vi "Ventilador2.vi"() -> ()   [LabVIEW 2019]
uses:
  <vilib>/Analysis/polynomials.llb/Polynomial Roots (DBL).vi
  <vilib>/Analysis/NI_AALPro.lvlib
panel:
  in  "Vertical Pointer Slide":dbl
  out "Aquisição pressão respiratória":dbl(graph)
  out "Válvula expiração":dbl(graph)
  in  "Pausa inspiração":dbl
  in  "Limite pressão inspiratória":dbl
  in  "OK Button":bool
  in  "Root 3":dbl
  in  "Root 2":dbl
  in  "Root 1":dbl
  in  "Incremento":dbl
  in  "Fluxo inicial":dbl
  in  "STOP":bool=TRUE
  out "Tempos de inspirações possíveis":cdb[](array[numeric])
  out "Tempo do ciclo respiratório":u32(graph)
  out "Válvula Inspiração":dbl(graph)
  in  "stop":bool
  in  "Tempo de respiração":dbl
  in  "Proporção Inspiração/respiração":string(combo)
  in  "Tempo corrido":dbl
  in  "Tipo de ventilação":string(combo)
  in  "Tipo de ciclo":string(combo)
  in  "Volume corrente":dbl
  in  "Tempo expiratório":dbl
  in  "Tempo inspiratório":dbl
  out "Fluxo respiratório medido":dbl
  in  "Frequência respiratória":dbl
  in  "Forma de onda":string(combo)
  in  "Fluxo respiratório set point":dbl
  # "rpm"
  # "(cmH2O)"
  # "(s)"
  # "\"Pausa inspiração\" neste programa está funcionando\ntambém como tempo de inspiração \ntotal, dado que não temos ainda nem \no controle nem a estimativa da rampa \nde subida da pressão do pulmão do paciente\npara diferenciar os valores"
  # "\"Vertical Pointer Slide\" está simulando a pressão\nno pulmão do paciente, você deve\n setá-lo para o valor de \"Limite pressão \ninspiratória\" quando Válvula inspiração =1 (aberta) e \nVálvula expiração = 0 (fechada) e para 0 (ou um valor \ndiferente de \"Limite pressão Inspiratória\") quando \nVálvula inspiração = 0 (fechada) e  Válvula expiração = 1 \n(aberta) para simular o ciclo de respiração natural."
  # "(s)"
  # "(s)"
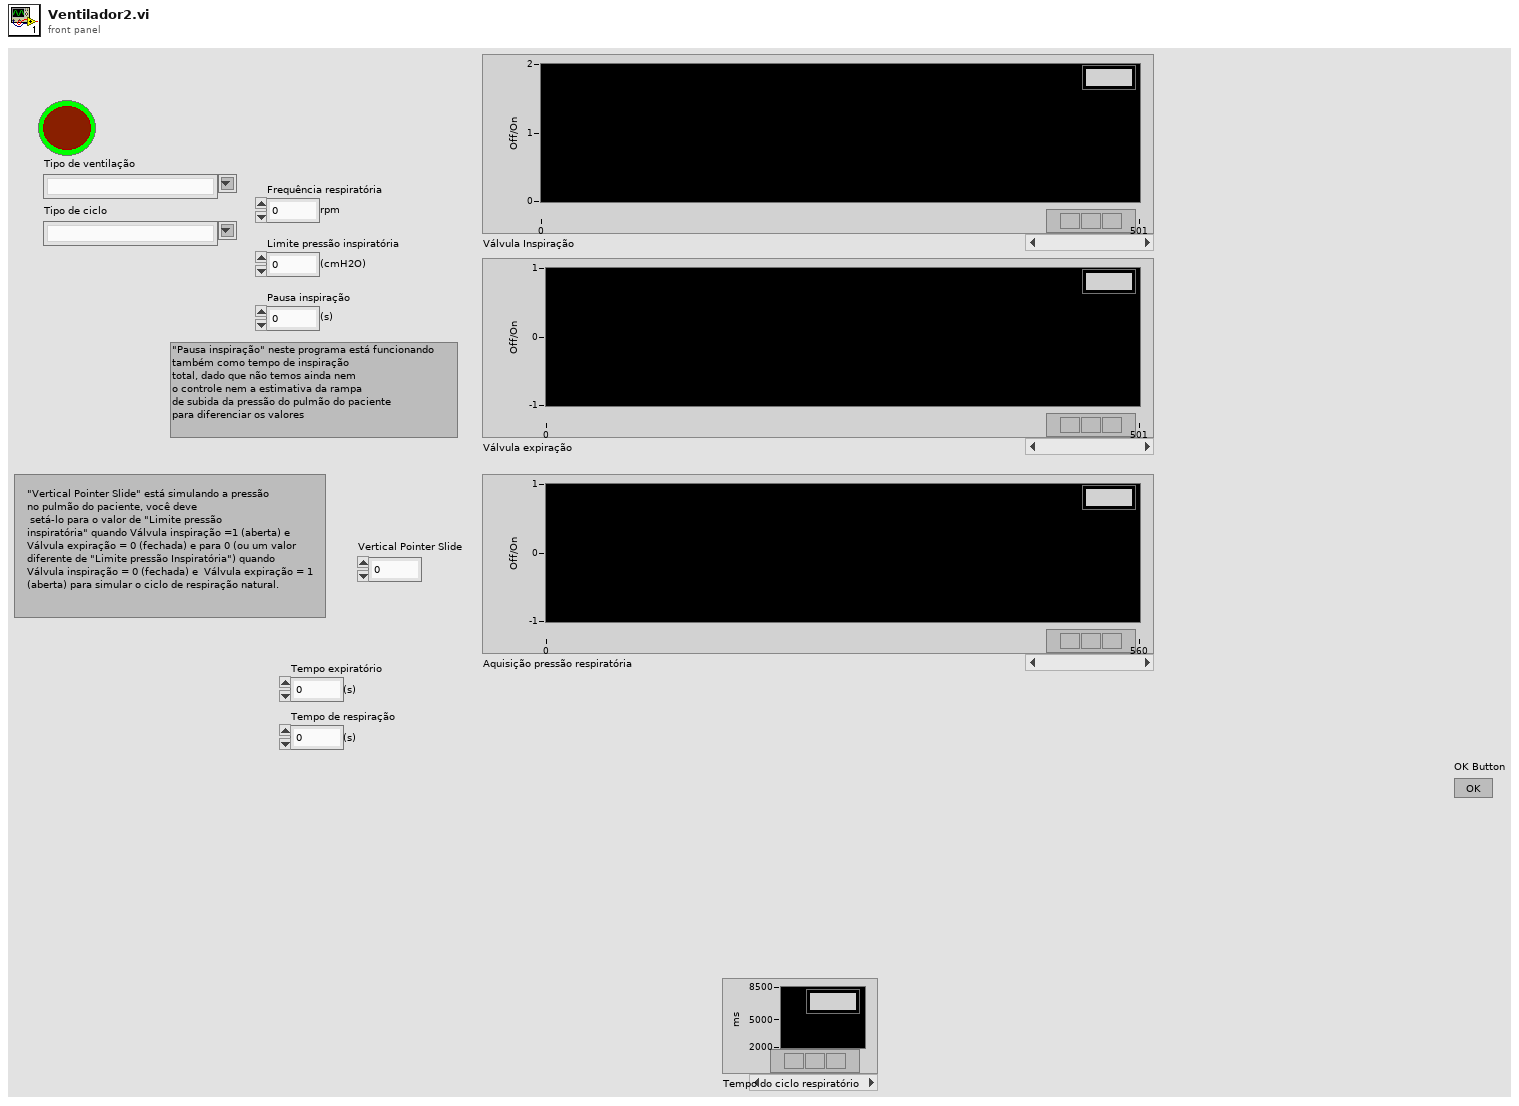
[diagram p1: front panel]
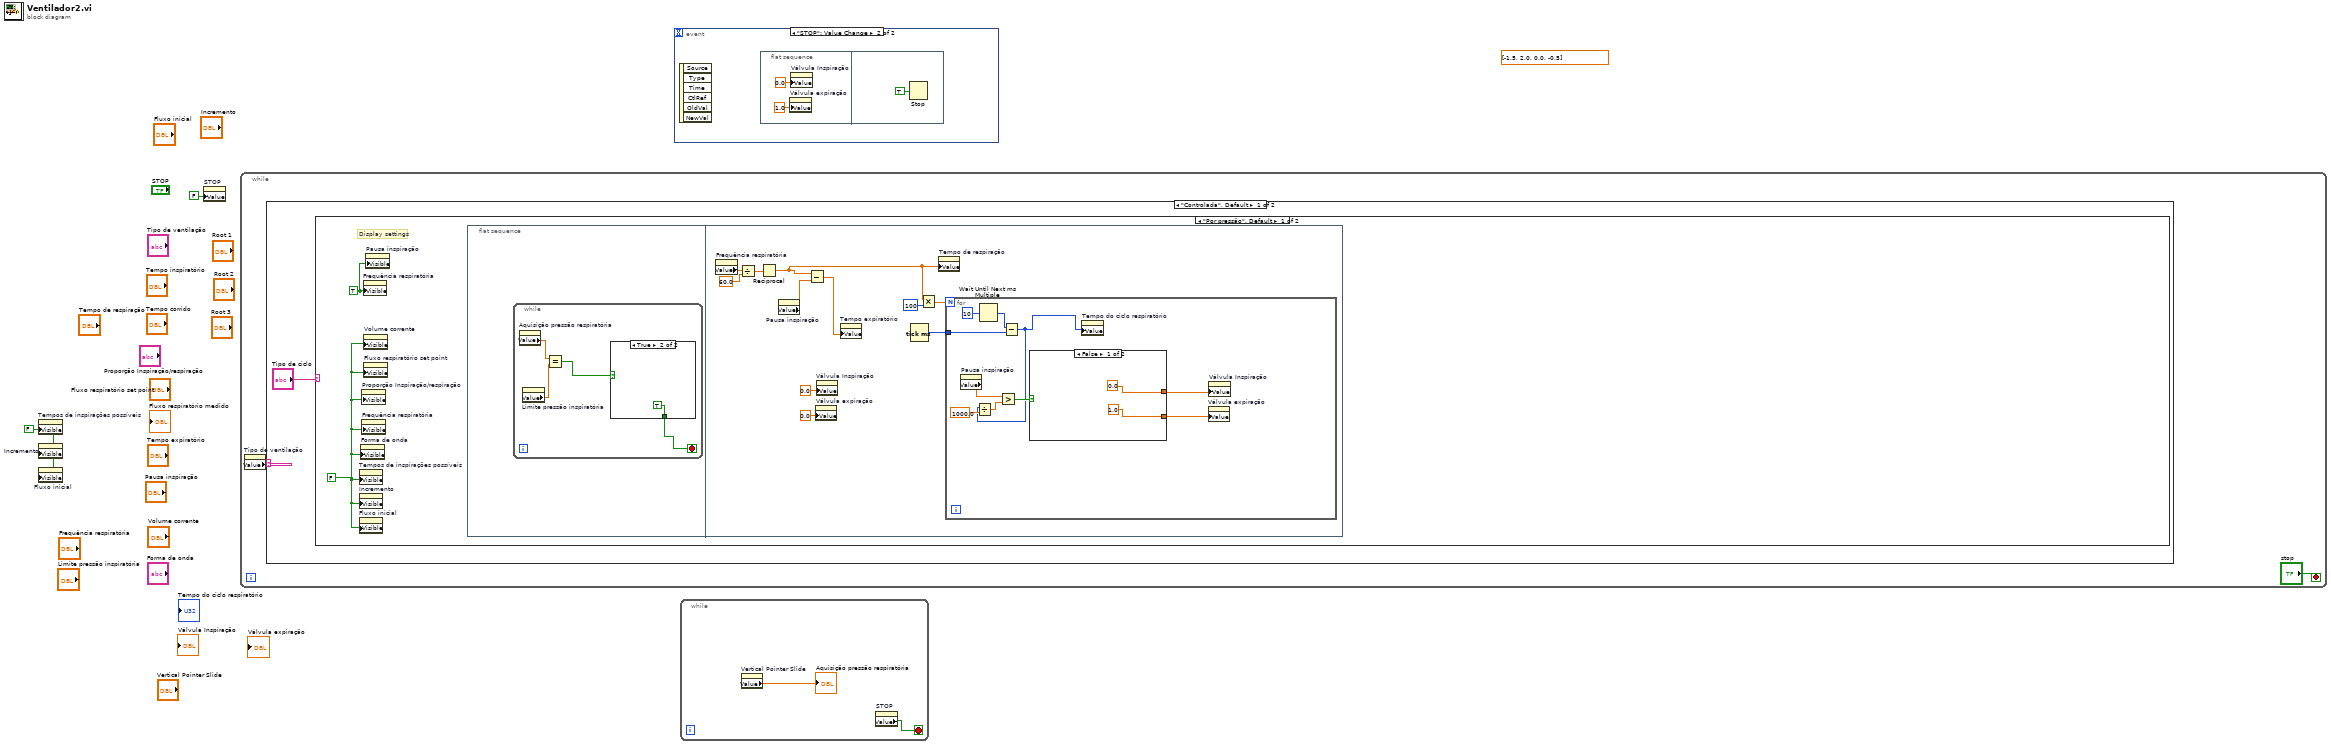
[diagram p0: block diagram]
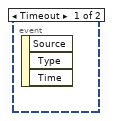
[diagram p2: hidden frame]
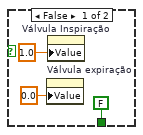
[diagram p3: hidden frame]
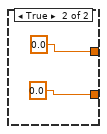
[diagram p4: hidden frame]
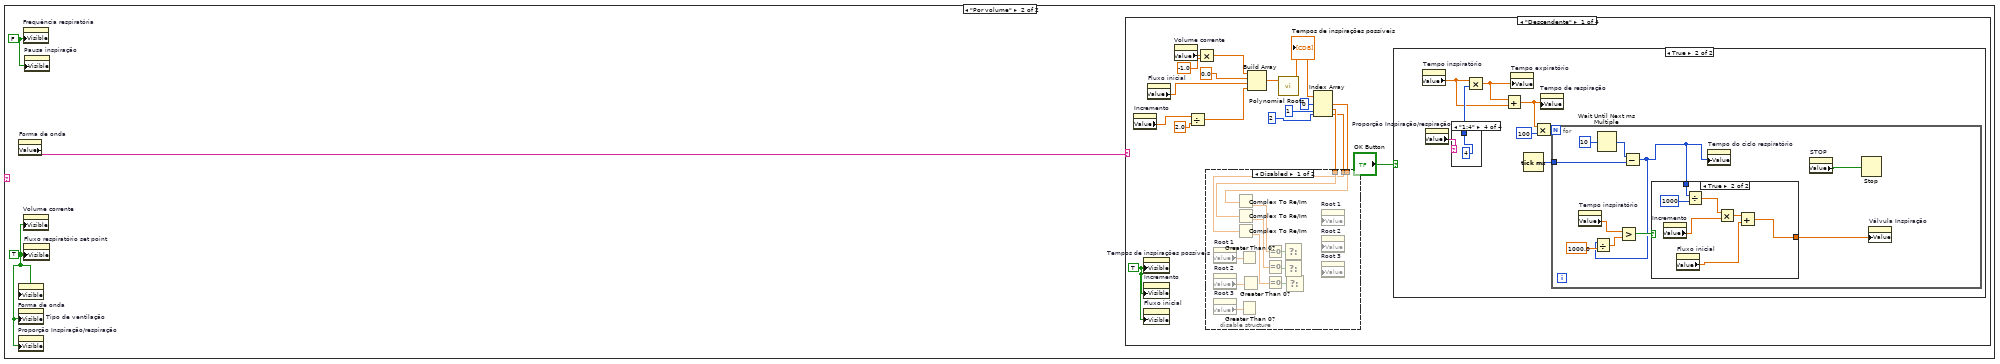
[diagram p5: hidden frame]
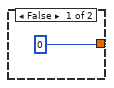
[diagram p8: hidden frame]
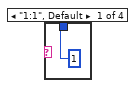
[diagram p9: hidden frame]
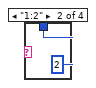
[diagram p10: hidden frame]
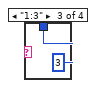
[diagram p11: hidden frame]
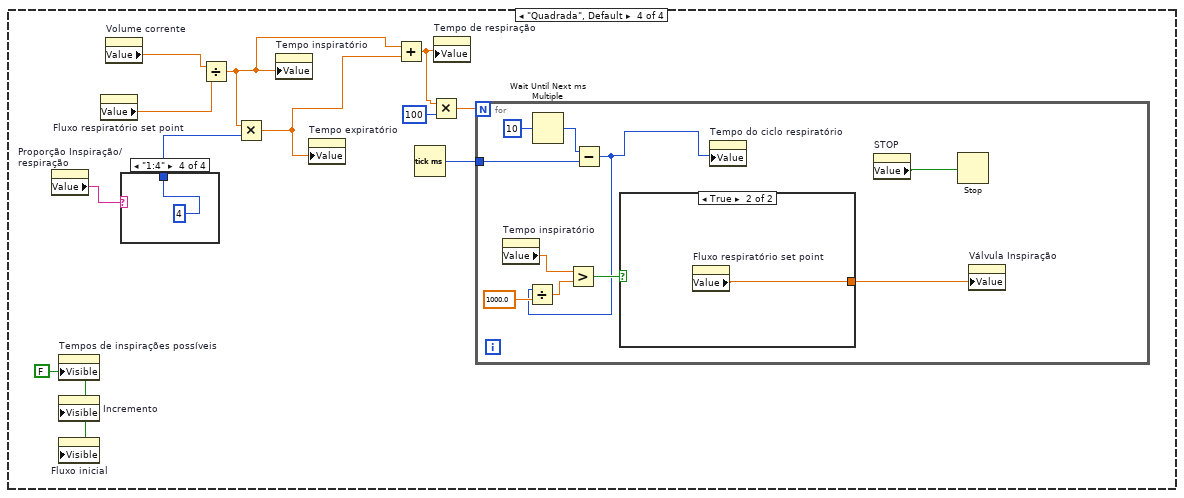
[diagram p14: hidden frame]
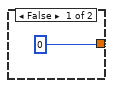
[diagram p15: hidden frame]
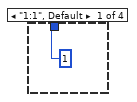
[diagram p16: hidden frame]
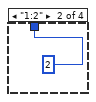
[diagram p17: hidden frame]
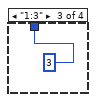
[diagram p18: hidden frame]
diagram:
  w1 = FALSE ("Visible")
  (unwired) dbl[] [-1.5, 2.0, 0.0, -0.5] ("P(x)")
  n1 = property on="Tempos de inspirações possíveis" class="Arr (strict)"("Visible"=w1) -> ()  [unwired: 2 in, 2 out]
  n2 = property on="Incremento" class="DigNum (strict)"("Visible"=w1) -> ()  [unwired: 2 in, 2 out]
  n3 = property on="Fluxo inicial" class="DigNum (strict)"("Visible"=w1) -> ()  [unwired: 2 in, 2 out]
  n4 = property on="STOP" class="Bool (strict)"("Value"=FALSE ("STOP")) -> ()  [unwired: 2 in, 2 out]
  n5 = while {
    stop <- "stop" stop-if-true
    n6 = property on="Tipo de ventilação" class="CmbBox"() -> ("Value"=w4:string)  [unwired: 2 in, 2 out]
    n7 = case shown="\"Controlada\", Default" w4 {
      frame "Controlada", Default {
        n8 = case shown="\"Por pressão\", Default" "Tipo de ciclo" {
          frame "Por pressão", Default {
            w6 = TRUE ("Visible")
            w7 = FALSE ("Visible")
            # "Display settings"
            n9 = property on="Tempos de inspirações possíveis" class="Arr (strict)"("Visible"=w7) -> ()  [unwired: 2 in, 2 out]
            n10 = property on="Incremento" class="DigNum (strict)"("Visible"=w7) -> ()  [unwired: 2 in, 2 out]
            n11 = property on="Fluxo inicial" class="DigNum (strict)"("Visible"=w7) -> ()  [unwired: 2 in, 2 out]
            n12 = property on="Forma de onda" class="CmbBox"("Visible"=w7) -> ()  [unwired: 2 in, 2 out]
            n13 = property on="Proporção Inspiração/respiração" class="CmbBox"("Visible"=w7) -> ()  [unwired: 2 in, 2 out]
            n14 = property on="Frequência respiratória" class="DigNum (strict)"("Visible"=w7) -> ()  [unwired: 2 in, 2 out]
            n15 = property on="Frequência respiratória" class="DigNum (strict)"("Visible"=w6) -> ()  [unwired: 2 in, 2 out]
            n16 = property on="Volume corrente" class="DigNum (strict)"("Visible"=w7) -> ()  [unwired: 2 in, 2 out]
            n17 = property on="Fluxo respiratório set point" class="DigNum (strict)"("Visible"=w7) -> ()  [unwired: 2 in, 2 out]
            n18 = property on="Pausa inspiração" class="DigNum (strict)"("Visible"=w6) -> ()  [unwired: 2 in, 2 out]
            n19 = flat-sequence {
              frame #0 {
                n20 = while {
                  stop <- w8 stop-if-true
                  n21 = property on="Aquisição pressão respiratória" class="WFChart (strict)"() -> ("Value"=w9:dbl)  [unwired: 2 in, 2 out]
                  n22 = property on="Limite pressão inspiratória" class="DigNum (strict)"() -> ("Value"=w11:dbl)  [unwired: 2 in, 2 out]
                  n23 = Equal?(x=w9, y=w11) -> (x = y?=w10:bool)
                  n24 = case shown="True" w10 {
                    tunnel: [FALSE TRUE] -> w8
                    frame False {
                      n25 = property on="Válvula expiração" class="WFChart (strict)"("Value"=0.0 ("Válvula expiração")) -> ()  [unwired: 2 in, 2 out]
                      n26 = property on="Válvula Inspiração" class="WFChart (strict)"("Value"=1.0 ("Válvula Inspiração")) -> ()  [unwired: 2 in, 2 out]
                    }
                    frame True {
                    }
                  }
                }
              }
              frame #1 {
                n27 = property on="Frequência respiratória" class="DigNum (strict)"() -> ("Value"=w23:dbl)  [unwired: 2 in, 2 out]
                n28 = Divide(x=w23, y=60.0) -> (x/y=w24:dbl)
                n29 = Reciprocal(x=w24) -> (1/x=w16:dbl)
                n30 = property on="Pausa inspiração" class="DigNum (strict)"() -> ("Value"=w25:dbl)  [unwired: 2 in, 2 out]
                n31 = Subtract(x=w16, y=w25) -> (x-y=w26:dbl)
                n32 = property on="Válvula expiração" class="WFChart (strict)"("Value"=0.0 ("Válvula expiração")) -> ()  [unwired: 2 in, 2 out]
                n33 = property on="Válvula Inspiração" class="WFChart (strict)"("Value"=0.0 ("Válvula Inspiração")) -> ()  [unwired: 2 in, 2 out]
                n34 = property on="Tempo expiratório" class="DigNum (strict)"("Value"=w26) -> ()  [unwired: 2 in, 2 out]
                n35 = Tick Count (ms)() -> (millisecond timer value=w21:u32)
                n36 = Multiply(x=w16, y=100) -> (x*y=w22:dbl)
                n37 = property on="Tempo de respiração" class="DigNum (strict)"("Value"=w16) -> ()  [unwired: 2 in, 2 out]
                n38 = for {
                  N: w22 -> [_]
                  tunnel: w21 -> [w34]
                  n39 = property on="Pausa inspiração" class="DigNum (strict)"() -> ("Value"=w32:dbl)  [unwired: 2 in, 2 out]
                  n40 = Wait Until Next ms Multiple(millisecond multiple=u32 10) -> (millisecond timer value=w36:u32)
                  n41 = Subtract(x=w36, y=w34) -> (x-y=w29:u32)
                  n42 = Divide(x=w29, y=1000.0) -> (x/y=w31:dbl)
                  n43 = Greater?(x=w32, y=w31) -> (0:w33:bool)
                  n44 = case shown="False" w33 {
                    tunnel: [0.0 ("Válvula Inspiração") 0.0 ("y")] -> w28
                    tunnel: [1.0 ("Válvula expiração") 0.0 ("y")] -> w27
                    frame False {
                    }
                    frame True {
                    }
                  }
                  n45 = property on="Tempo do ciclo respiratório" class="WFChart (strict)"("Value"=w29) -> ()  [unwired: 2 in, 2 out]
                  n46 = property on="Válvula expiração" class="WFChart (strict)"("Value"=w27) -> ()  [unwired: 2 in, 2 out]
                  n47 = property on="Válvula Inspiração" class="WFChart (strict)"("Value"=w28) -> ()  [unwired: 2 in, 2 out]
                }
              }
            }
          }
          frame "Por volume" {
            w41 = FALSE ("Visible")
            w42 = TRUE ("Visible")
            n48 = property on="Forma de onda" class="CmbBox"("Visible"=w42) -> ()  [unwired: 2 in, 2 out]
            n49 = property on="Tipo de ventilação" class="CmbBox"("Visible"=w42) -> ()  [unwired: 2 in, 2 out]
            n50 = property on="Proporção Inspiração/respiração" class="CmbBox"("Visible"=w42) -> ()  [unwired: 2 in, 2 out]
            n51 = property on="Forma de onda" class="CmbBox"() -> ("Value"=w43:string)  [unwired: 2 in, 2 out]
            n52 = property on="Frequência respiratória" class="DigNum (strict)"("Visible"=w41) -> ()  [unwired: 2 in, 2 out]
            n53 = property on="Volume corrente" class="DigNum (strict)"("Visible"=w42) -> ()  [unwired: 2 in, 2 out]
            n54 = property on="Fluxo respiratório set point" class="DigNum (strict)"("Visible"=w42) -> ()  [unwired: 2 in, 2 out]
            n55 = property on="Pausa inspiração" class="DigNum (strict)"("Visible"=w41) -> ()  [unwired: 2 in, 2 out]
            n56 = case shown="\"Descendente\"" w43 {
              frame "Descendente" {
                w44 = TRUE ("Visible")
                n57 = property on="Incremento" class="DigNum (strict)"() -> ("Value"=w60:dbl)  [unwired: 2 in, 2 out]
                n58 = property on="Tempos de inspirações possíveis" class="Arr (strict)"("Visible"=w44) -> ()  [unwired: 2 in, 2 out]
                n59 = property on="Incremento" class="DigNum (strict)"("Visible"=w44) -> ()  [unwired: 2 in, 2 out]
                n60 = property on="Fluxo inicial" class="DigNum (strict)"("Visible"=w44) -> ()  [unwired: 2 in, 2 out]
                n61 = property on="Fluxo inicial" class="DigNum (strict)"() -> ("Value"=w49:dbl)  [unwired: 2 in, 2 out]
                n62 = property on="Volume corrente" class="DigNum (strict)"() -> ("Value"=w59:dbl)  [unwired: 2 in, 2 out]
                n63 = Divide(x=w60, y=2.0) -> (x/y=w48:dbl)
                n64 = Multiply(x=w59, y=-1.0) -> (x*y=w51:dbl)
                n65 = Build Array(w51, 0.0 ("element"), w49, w48) -> (w47:dbl[])
                n66 = call-poly <vilib>:"Polynomial Roots.vi"("P(x)"=w47) -> ("Roots"=w61:cdb[])  [unwired: 9 in, 1 out]
                "Tempos de inspirações possíveis" <- w61
                n67 = Index Array(array=w61, index #1=0 ("index"), index #2=1 ("index"), index #3=2 ("index")) -> (element #1=w46:cdb, element #2=w53:cdb, element #3=w52:cdb)
                n68 = disable-structure shown="Disabled" {
                  disable-tunnel: w53 -> [w73 _]
                  disable-tunnel: w52 -> [w72 _]
                  disable-tunnel: w46 -> [w71 _]
                  frame Disabled {
                    n69 = property on="Root 1" class="DigNum (strict)"() -> ("Value"=w70:dbl)  [unwired: 2 in, 2 out]
                    n70 = property on="Root 2" class="DigNum (strict)"() -> ("Value"=w69:dbl)  [unwired: 2 in, 2 out]
                    n71 = property on="Root 3" class="DigNum (strict)"() -> ("Value"=w68:dbl)  [unwired: 2 in, 2 out]
                    n72 = Complex To Re/Im(x + iy=w71) -> (y=w65:dbl)  [unwired: 1 out]
                    n73 = Complex To Re/Im(x + iy=w73) -> (y=w66:dbl)  [unwired: 1 out]
                    n74 = Complex To Re/Im(x + iy=w72) -> (y=w67:dbl)  [unwired: 1 out]
                    n75 = Greater Than 0?(x=w70) -> ()  [unwired: 1 out]
                    n76 = Greater Than 0?(x=w68) -> ()  [unwired: 1 out]
                    n77 = Greater Than 0?(x=w69) -> ()  [unwired: 1 out]
                    n78 = Equal To 0?(x=w65) -> (x = 0?=w64:bool)
                    n79 = Equal To 0?(x=w66) -> (x = 0?=w63:bool)
                    n80 = Equal To 0?(x=w67) -> (x = 0?=w62:bool)
                    n81 = Select(s=w64) -> ()  [unwired: 2 in, 1 out]
                    n82 = Select(s=w63) -> ()  [unwired: 2 in, 1 out]
                    n83 = Select(s=w62) -> ()  [unwired: 2 in, 1 out]
                    n84 = property on="Root 1" class="DigNum (strict)" props=["Value"]() -> ()  [unwired: 3 in, 2 out]
                    n85 = property on="Root 2" class="DigNum (strict)" props=["Value"]() -> ()  [unwired: 3 in, 2 out]
                    n86 = property on="Root 3" class="DigNum (strict)" props=["Value"]() -> ()  [unwired: 3 in, 2 out]
                  }
                  frame Enabled {
                  }
                }
                n87 = case shown="True" "OK Button" {
                  frame False {
                  }
                  frame True {
                    n88 = property on="Tempo inspiratório" class="DigNum (strict)"() -> ("Value"=w75:dbl)  [unwired: 2 in, 2 out]
                    n89 = property on="Proporção Inspiração/respiração" class="CmbBox"() -> ("Value"=w81:string)  [unwired: 2 in, 2 out]
                    n90 = case shown="\"1:4\"" w81 {
                      tunnel: [1 2 3 4] -> w77
                      frame "1:1", Default {
                      }
                      frame "1:2" {
                      }
                      frame "1:3" {
                      }
                      frame "1:4" {
                      }
                    }
                    n91 = Multiply(x=w75, y=w77) -> (x*y=w76:dbl)
                    n92 = Add(x=w76, y=w75) -> (x+y=w74:dbl)
                    n93 = property on="Tempo expiratório" class="DigNum (strict)"("Value"=w76) -> ()  [unwired: 2 in, 2 out]
                    n94 = Tick Count (ms)() -> (millisecond timer value=w80:u32)
                    n95 = Multiply(x=w74, y=100) -> (x*y=w79:dbl)
                    n96 = property on="Tempo de respiração" class="DigNum (strict)"("Value"=w74) -> ()  [unwired: 2 in, 2 out]
                    n97 = for {
                      N: w79 -> [_]
                      tunnel: w80 -> [w89]
                      n98 = property on="Tempo inspiratório" class="DigNum (strict)"() -> ("Value"=w87:dbl)  [unwired: 2 in, 2 out]
                      n99 = Wait Until Next ms Multiple(millisecond multiple=u32 10) -> (millisecond timer value=w91:u32)
                      n100 = Subtract(x=w91, y=w89) -> (x-y=w83:u32)
                      n101 = Divide(x=w83, y=1000.0) -> (x/y=w86:dbl)
                      n102 = Greater?(x=w87, y=w86) -> (0:w88:bool)
                      n103 = case shown="True" w88 {
                        tunnel: [0 w94] -> w82
                        tunnel: w83 -> [_ w99]
                        frame False {
                        }
                        frame True {
                          n104 = property on="Incremento" class="DigNum (strict)"() -> ("Value"=w96:dbl)  [unwired: 2 in, 2 out]
                          n105 = property on="Fluxo inicial" class="DigNum (strict)"() -> ("Value"=w93:dbl)  [unwired: 2 in, 2 out]
                          n106 = Divide(x=w99, y=u32 1000) -> (x/y=w97:dbl)
                          n107 = Multiply(x=w97, y=w96) -> (x*y=w95:dbl)
                          n108 = Add(x=w95, y=w93) -> (x+y=w94:dbl)
                        }
                      }
                      n109 = property on="Tempo do ciclo respiratório" class="WFChart (strict)"("Value"=w83) -> ()  [unwired: 2 in, 2 out]
                      n110 = property on="STOP" class="Bool (strict)"() -> ("Value"=w84:bool)  [unwired: 2 in, 2 out]
                      n111 = Stop(stop? (T)=w84) -> ()
                      n112 = property on="Válvula Inspiração" class="WFChart (strict)"("Value"=w82) -> ()  [unwired: 2 in, 2 out]
                    }
                  }
                }
              }
              frame "Ascendente" {
              }
              frame "Sinusoidal" {
              }
              frame "Quadrada", Default {
                w104 = FALSE ("Visible")
                n113 = property on="Proporção Inspiração/respiração" class="CmbBox"() -> ("Value"=w112:string)  [unwired: 2 in, 2 out]
                n114 = property on="Tempos de inspirações possíveis" class="Arr (strict)"("Visible"=w104) -> ()  [unwired: 2 in, 2 out]
                n115 = property on="Incremento" class="DigNum (strict)"("Visible"=w104) -> ()  [unwired: 2 in, 2 out]
                n116 = property on="Fluxo inicial" class="DigNum (strict)"("Visible"=w104) -> ()  [unwired: 2 in, 2 out]
                n117 = property on="Fluxo respiratório set point" class="DigNum (strict)"() -> ("Value"=w114:dbl)  [unwired: 2 in, 2 out]
                n118 = property on="Volume corrente" class="DigNum (strict)"() -> ("Value"=w113:dbl)  [unwired: 2 in, 2 out]
                n119 = case shown="\"1:4\"" w112 {
                  tunnel: [1 2 3 4] -> w111
                  frame "1:1", Default {
                  }
                  frame "1:2" {
                  }
                  frame "1:3" {
                  }
                  frame "1:4" {
                  }
                }
                n120 = Divide(x=w113, y=w114) -> (x/y=w108:dbl)
                n121 = Multiply(x=w108, y=w111) -> (x*y=w107:dbl)
                n122 = property on="Tempo inspiratório" class="DigNum (strict)"("Value"=w108) -> ()  [unwired: 2 in, 2 out]
                n123 = property on="Tempo expiratório" class="DigNum (strict)"("Value"=w107) -> ()  [unwired: 2 in, 2 out]
                n124 = Add(x=w108, y=w107) -> (x+y=w106:dbl)
                n125 = Tick Count (ms)() -> (millisecond timer value=w110:u32)
                n126 = Multiply(x=w106, y=100) -> (x*y=w109:dbl)
                n127 = property on="Tempo de respiração" class="DigNum (strict)"("Value"=w106) -> ()  [unwired: 2 in, 2 out]
                n128 = for {
                  N: w109 -> [_]
                  tunnel: w110 -> [w122]
                  n129 = property on="Tempo inspiratório" class="DigNum (strict)"() -> ("Value"=w120:dbl)  [unwired: 2 in, 2 out]
                  n130 = Wait Until Next ms Multiple(millisecond multiple=u32 10) -> (millisecond timer value=w124:u32)
                  n131 = Subtract(x=w124, y=w122) -> (x-y=w117:u32)
                  n132 = Divide(x=w117, y=1000.0) -> (x/y=w119:dbl)
                  n133 = Greater?(x=w120, y=w119) -> (0:w121:bool)
                  n134 = case shown="True" w121 {
                    tunnel: [0 w126] -> w116
                    frame False {
                    }
                    frame True {
                      n135 = property on="Fluxo respiratório set point" class="DigNum (strict)"() -> ("Value"=w126:dbl)  [unwired: 2 in, 2 out]
                    }
                  }
                  n136 = property on="Tempo do ciclo respiratório" class="WFChart (strict)"("Value"=w117) -> ()  [unwired: 2 in, 2 out]
                  n137 = property on="STOP" class="Bool (strict)"() -> ("Value"=w115:bool)  [unwired: 2 in, 2 out]
                  n138 = Stop(stop? (T)=w115) -> ()
                  n139 = property on="Válvula Inspiração" class="WFChart (strict)"("Value"=w116) -> ()  [unwired: 2 in, 2 out]
                }
              }
            }
          }
        }
      }
      frame "Expontânea/Assistida" {
      }
    }
  }
  n140 = event shown="[1] \"STOP\": Value Change" {
    selector: _ -> [_ _]
    dyn-events: _ -> [_ _]
    timeout: _ -> [_ _]
    event Timeout {
      n141 = event-data() -> ()  [unwired: 1 in, 3 out]
    }
    event "STOP": Value Change {
      n142 = event-data() -> ()  [unwired: 1 in, 6 out]
      n143 = flat-sequence {
        frame #0 {
          n144 = property on="Válvula expiração" class="WFChart (strict)"("Value"=1.0 ("Válvula expiração")) -> ()  [unwired: 2 in, 2 out]
          n145 = property on="Válvula Inspiração" class="WFChart (strict)"("Value"=0.0 ("Válvula Inspiração")) -> ()  [unwired: 2 in, 2 out]
        }
        frame #1 {
          n146 = Stop(stop? (T)=TRUE) -> ()
        }
      }
    }
  }
  n147 = while {
    stop <- w135 stop-if-true
    n148 = property on="Vertical Pointer Slide" class="DigNum (strict)"() -> ("Value"=→"Aquisição pressão respiratória":dbl)  [unwired: 2 in, 2 out]
    n149 = property on="STOP" class="Bool (strict)"() -> ("Value"=w135:bool)  [unwired: 2 in, 2 out]
  }
